vi "Get API.vi"(8 "error in (no error)":errorcluster, 11 "Sequencer in":refnum<class "Sequencer.lvclass">) -> (0 "error out":errorcluster, 2 "API":string[](array[string]), 3 "Sequencer out":refnum<class "Sequencer.lvclass">)   [LabVIEW 2024, in "Ramses Sequencer.lvlib" / "Sequencer.lvclass"]
uses:
  Sequencer.lvclass
  Program Files (x86)/Enterative/Ramses Framework/Ramses Framework.lvlibp/Service/Service.lvclass
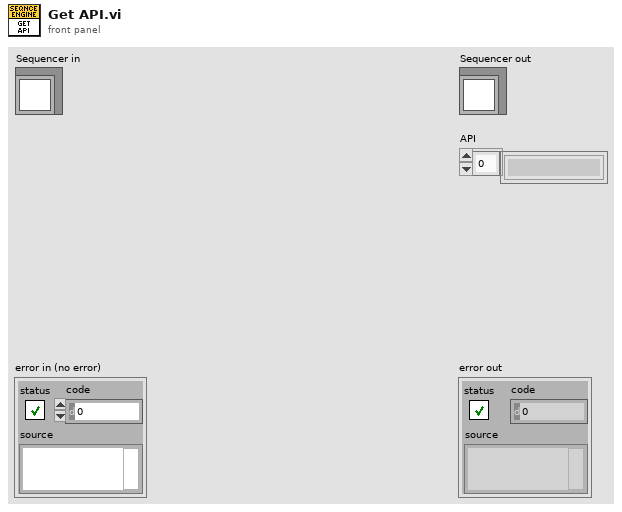
[diagram p1: front panel]
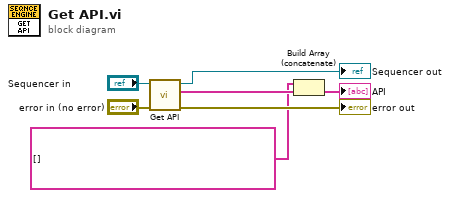
[diagram p0: block diagram]
diagram:
  n1 = call-parent "Get API.vi"("error in (no error)"="error in (no error)", "Service in"="Sequencer in") -> ("error out"=→"error out":errorcluster, "API"=w2:string[], "Service out"=→"Sequencer out":refnum<class "Sequencer.lvclass">)  [unwired: 7 in]
  n2 = Build Array (concatenate)(string[] [], w2) -> (→"API":string[])
